vi "Scan.vi"(11 "OT3IScan In":refnum<class "OT3IScan.lvclass">) -> (3 "OT3IScan Out":refnum<class "OT3IScan.lvclass">)   [LabVIEW 2018, in "OfficeTron3000.lvlib" / "OT3IScan.lvclass"]
uses:
  OT3IScan.lvclass
  OfficeTron3000/OfficeTron3000.lvclass
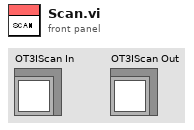
[diagram p1: front panel]
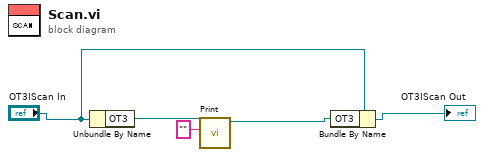
[diagram p0: block diagram]
diagram:
  n1 = Unbundle By Name("OT3IScan In") -> ("OT3"=w3:refnum<class "OfficeTron3000.lvclass">)
  n2 = call "Print.vi"("String"="", "OfficeTron3000 In"=w3) -> ("OfficeTron3000 Out"=w2:refnum<class "OfficeTron3000.lvclass">)  [unwired: 9 in]
  n3 = Bundle By Name(cluster="OT3IScan In", "OT3"=w2) -> (→"OT3IScan Out":refnum<class "OT3IScan.lvclass">)
